vi "Open.vi"(8 "error in (no error)":errorcluster, 11 "Reference Control in":refnum<class "Reference Control.lvclass">) -> (0 "error out":errorcluster, 3 "Reference Control out":refnum<class "Reference Control.lvclass">)   [LabVIEW 2016, in "Reference Control.lvclass"]
uses:
  Reference Control.lvclass
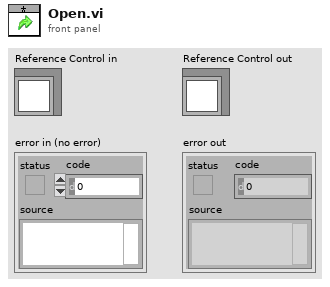
[diagram p1: front panel]
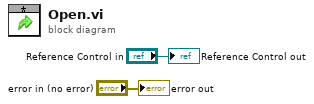
[diagram p0: block diagram]
diagram:
  "error out" <- "error in (no error)"
  "Reference Control out" <- "Reference Control in"
